vi "BuvCtrlVI.vi"() -> ()   [LabVIEW 2013]
panel:
  out "SetVstr":string
  out "stop":bool=TRUE
  out "ErrMessage":string=" INSTRUCTIONS:\r\rNormal Use:  When using subVIs that incorporate the error in/error out (or error I/O) structure, place this handler where you want to inform the user of an error, typically at the end of the I/O data path, as the last action of the program.  If the error in error? is ERROR, the handler creates a message describing the error and its source.  If the type of dialog = 1 (default), the message is displayed to the user, who can only acknowedge it.  If the type = 2, the user can acknowledge the message or abort execution; aborting a program with active I/O is not recommended.  If the type = 0, no message is displayed; this is used to process the error programmatically, and the error out cluster elements are wired to individual terminals for that reason.  \r\rOther Use:\n\r\nlocal testing.  To test the error code of a subVI or function that does not have the error I/O structure, you can wire its error code and a source string to the local error code and error source inputs.  If error in error? indicates no error and error code is not equal to 0, the local code and source are substituted for the error in values, and error? is set TRUE (ERROR)."
  in  "TCP disconnect":bool
  out "connection ID":refnum<k5>
  out "_TCP disconnect":bool
  out "Active_num":i16
  out "ReadI":string
  out "status cluster":cluster{bool, bool, bool}
  in  "SetOutOFF":bool
  in  "error in":errorcluster
  out "errorOut":errorcluster
  in  "SetOutON":bool
  in  "SetVoltage":dbl format="%#.3g"
  in  "SetV":bool
  out "Active":bool
  in  "IP":string="0"
  out "ReadV":string
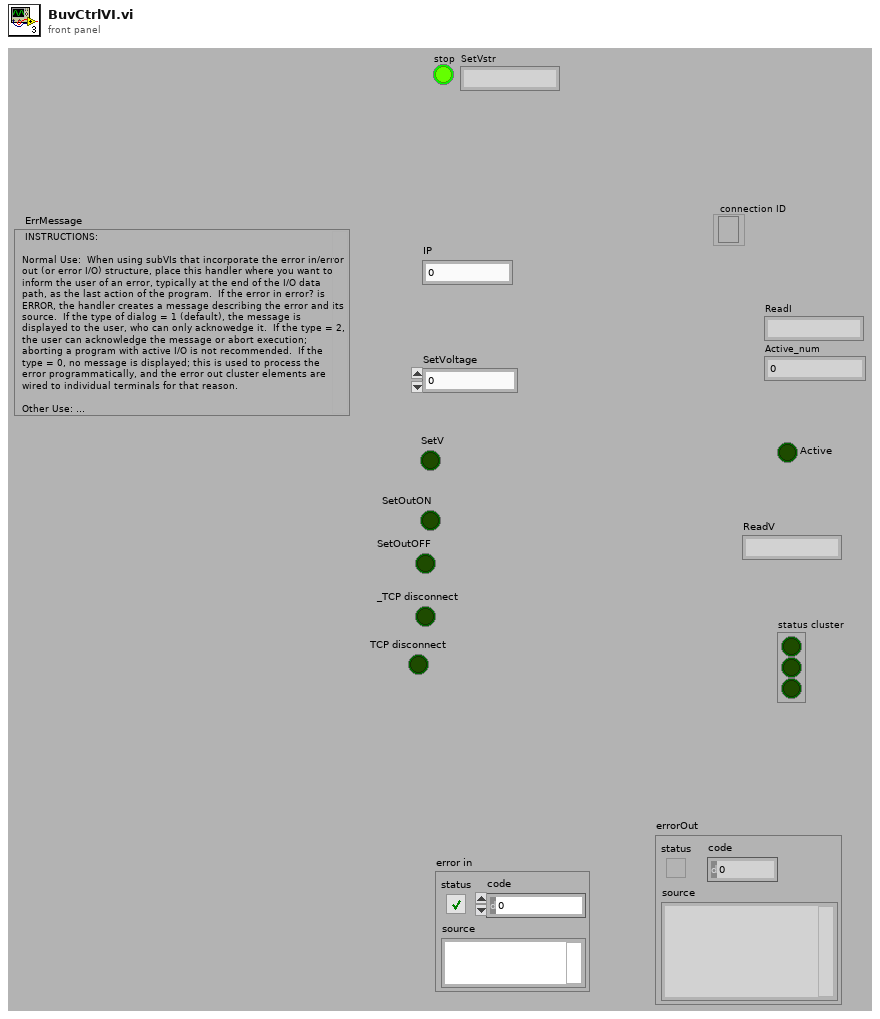
[diagram p1: front panel]
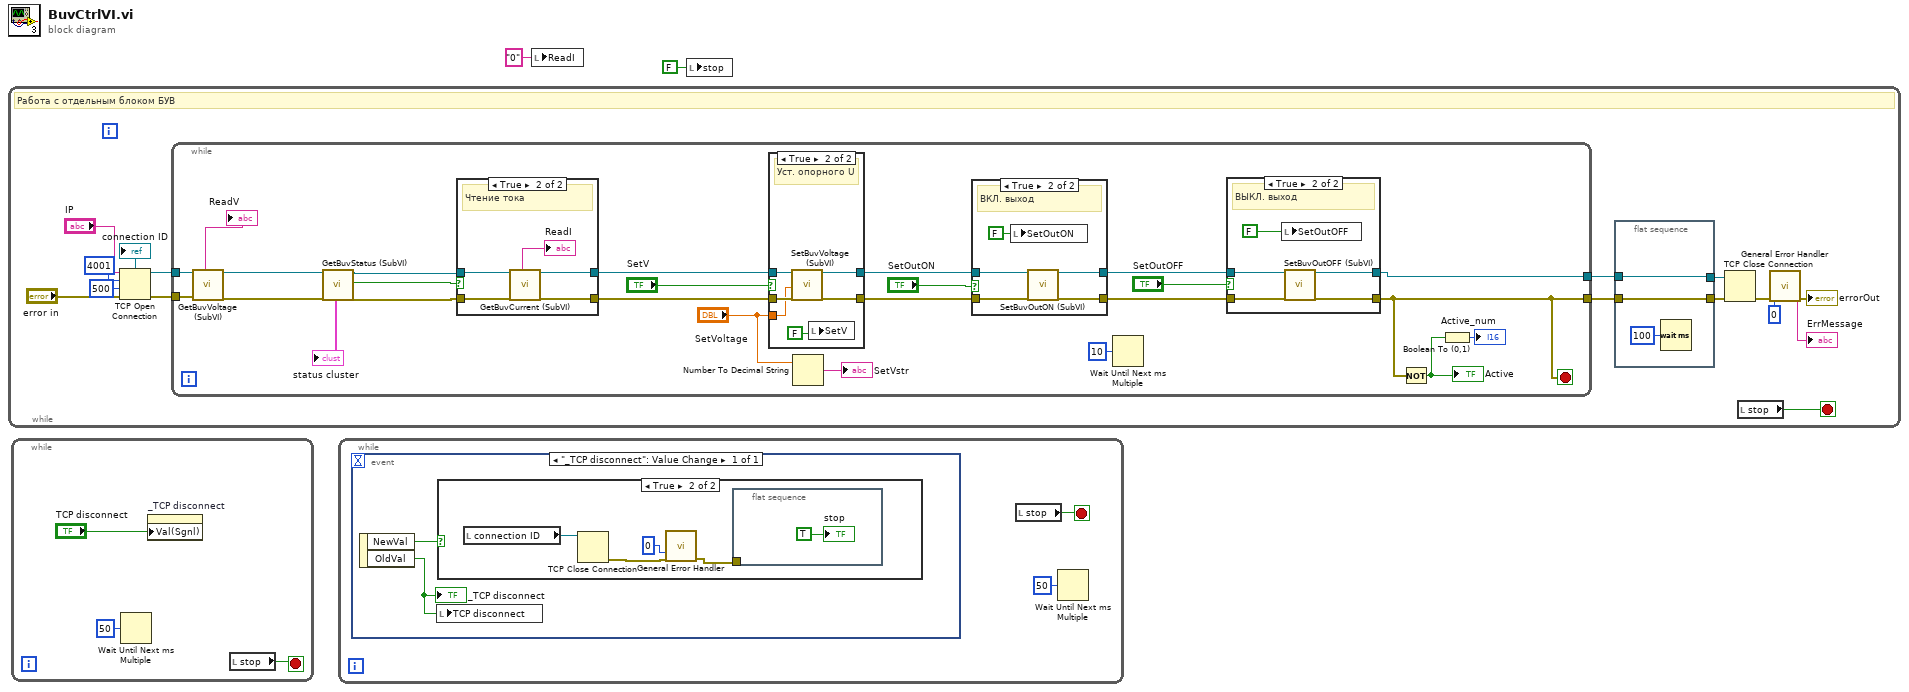
[diagram p0: block diagram]
diagram:
  n1 = while {
    stop <- w3 stop-if-true
    # "Работа с отдельным блоком БУВ"
    n2 = TCP Open Connection(address="IP", remote port or service name=u16 4001 ("Port"), timeout ms (60000)=500, error in (no error)="error in") -> (connection ID=w14:refnum<k5>, error out=w8:errorcluster)  [unwired: 1 out]
    "connection ID" <- w14
    n3 = while {
      tunnel: w14 -> [w45]
      tunnel: [w44] -> w7
      tunnel: [w25] -> w5
      tunnel: w8 -> [w34]
      stop <- w25 stop-if-true
      n4 = call "GetBuvVoltage (SubVI).vi"("connection ID in"=w45, "error in"=w34) -> ("Voltage"=→"ReadV":string, "connection ID out"=w28:refnum<k5>, "error out"=w27:errorcluster)  [unwired: 15 in]
      n5 = call "GetBuvStatus (SubVI).vi"("connection ID in"=w28, "error in"=w27) -> ("status cluster"=→"status cluster":cluster{bool, bool, bool}, "connection ID out"=w23:refnum<k5>, "I Ready"=w21:bool, "error out"=w22:errorcluster)  [unwired: 14 in]
      n6 = case shown="True" w21 {
        tunnel: [w46 w51] -> w38
        tunnel: [w47 w50] -> w39
        tunnel: w23 -> [w47 w49]
        tunnel: w22 -> [w46 w52]
        frame False {
        }
        frame True {
          # "Чтение тока"
          n7 = call "GetBuvCurrent (SubVI).vi"("connection ID in"=w49, "error in"=w52) -> ("Buv I"=→"ReadI":string, "connection ID out"=w50:refnum<k5>, "error out"=w51:errorcluster)  [unwired: 15 in]
        }
      }
      n8 = case shown="True" "SetV" {
        tunnel: w38 -> [w68 w73]
        tunnel: w39 -> [w67 w72]
        tunnel: [w68 w71] -> w43
        tunnel: [w67 w70] -> w42
        tunnel: "SetVoltage" -> [_ w69]
        frame False {
        }
        frame True {
          # "Уст. опорного U"
          n9 = call "SetBuvVoltage (SubVI).vi"("connection ID in"=w72, "BuvV2set"=w69, "error in"=w73) -> ("connection ID out"=w70:refnum<k5>, "error out"=w71:errorcluster)  [unwired: 15 in]
          n10 = local write "SetV"(FALSE ("NeedToSetVoltage")) -> ()
        }
      }
      n11 = Number To Decimal String(number="SetVoltage") -> (decimal integer string=→"SetVstr":string)  [unwired: 1 in]
      n12 = case shown="True" "SetOutON" {
        tunnel: w43 -> [w60 w65]
        tunnel: w42 -> [w61 w64]
        tunnel: [w60 w63] -> w41
        tunnel: [w61 w62] -> w40
        frame False {
        }
        frame True {
          # "ВКЛ. выход"
          n13 = local write "SetOutON"(FALSE ("NeedToSetVoltage")) -> ()
          n14 = call "SetBuvOutON (SubVI).vi"("connection ID in"=w64, "error in"=w65) -> ("connection ID out"=w62:refnum<k5>, "error out"=w63:errorcluster)  [unwired: 16 in]
        }
      }
      n15 = Wait Until Next ms Multiple(millisecond multiple=u32 10) -> ()  [unwired: 1 out]
      n16 = case shown="True" "SetOutOFF" {
        tunnel: w41 -> [w53 w58]
        tunnel: w40 -> [w54 w57]
        tunnel: [w53 w56] -> w25
        tunnel: [w54 w55] -> w44
        frame False {
        }
        frame True {
          # "ВЫКЛ. выход"
          n17 = local write "SetOutOFF"(FALSE ("NeedToSetVoltage")) -> ()
          n18 = call "SetBuvOutOFF (SubVI).vi"("connection ID in"=w57, "error in"=w58) -> ("connection ID out"=w55:refnum<k5>, "error out"=w56:errorcluster)  [unwired: 16 in]
        }
      }
      n19 = Not(x=w25) -> (.not. x?=w33:bool)
      "Active" <- w33
      n20 = Boolean To (0,1)(Boolean=w33) -> (0, 1=→"Active_num":i16)
    }
    n21 = flat-sequence {
      tunnel: [w19] -> w6
      tunnel: w7 -> [w19]
      tunnel: w5 -> [w18]
      tunnel: [w18] -> w4
      frame #0 {
        n22 = Wait (ms)(milliseconds to wait=u32 100 ("millisecond multiple")) -> ()  [unwired: 1 out]
      }
    }
    n23 = TCP Close Connection(connection ID=w6, error in (no error)=w4) -> (error out=w10:errorcluster)  [unwired: 2 out]
    n24 = local read "stop"() -> (w3:bool)
    n25 = call <vilib>:"General Error Handler.vi"("type of dialog (OK msg:1)"=u32 0 ("millisecond multiple"), "error in (no error)"=w10) -> ("message"=→"ErrMessage":string, "error out"=→"errorOut":errorcluster)  [unwired: 9 in, 3 out]
  }
  n26 = while {
    stop <- w75 stop-if-true
    n27 = Wait Until Next ms Multiple(millisecond multiple=u32 50) -> ()  [unwired: 1 out]
    n28 = property on="_TCP disconnect" class="Bool (strict)"("Val(Sgnl)"="TCP disconnect") -> ()  [unwired: 2 in, 2 out]
    n29 = local read "stop"() -> (w75:bool)
  }
  n30 = while {
    stop <- w78 stop-if-true
    n31 = event shown="[0] \"_TCP disconnect\": Value Change" {
      selector: _ -> [_]
      dyn-events: _ -> [_]
      timeout: _ -> [_]
      event "_TCP disconnect": Value Change {
        n32 = event-data() -> ("NewVal"=w81:bool, "OldVal"=w80:bool)  [unwired: 1 in]
        "_TCP disconnect" <- w80
        n33 = local write "TCP disconnect"(w80) -> ()
        n34 = case shown="True" w81 {
          frame False {
          }
          frame True {
            n35 = local read "connection ID"() -> (w85:refnum<k5>)
            n36 = TCP Close Connection(connection ID=w85) -> (error out=w84:errorcluster)  [unwired: 1 in, 2 out]
            n37 = call <vilib>:"General Error Handler.vi"("type of dialog (OK msg:1)"=u32 0 ("millisecond multiple"), "error in (no error)"=w84) -> ("error out"=w82:errorcluster)  [unwired: 9 in, 4 out]
            n38 = flat-sequence {
              tunnel: w82 -> [_]
              frame #0 {
                "stop" <- TRUE ("stop? (T)")
              }
            }
          }
        }
      }
    }
    n39 = local read "stop"() -> (w78:bool)
    n40 = Wait Until Next ms Multiple(millisecond multiple=u32 50) -> ()  [unwired: 1 out]
  }
  n41 = local write "ReadI"("0" ("ReadI")) -> ()
  n42 = local write "stop"(FALSE ("stop")) -> ()
